vi "AfterZeroSpreadColor-V2.2.vi"(4 "BackMap":i32[][](array[numeric]), 5 "WhichPlayer":i32, 6 "Position":i32[][](array[numeric])=[[0, 1], [1, 0]]) -> (0 "col":i32, 1 "row":i32, 2 "Numeric":dbl)   [LabVIEW 2014]
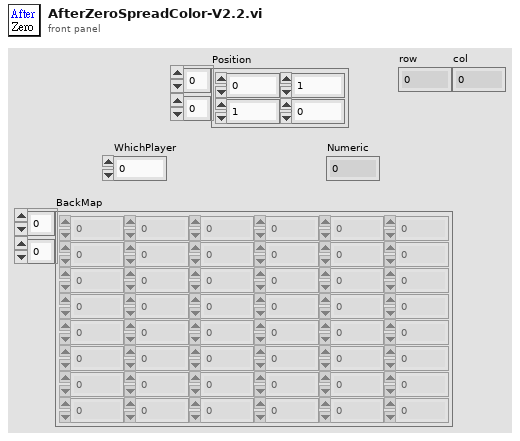
[diagram p1: front panel]
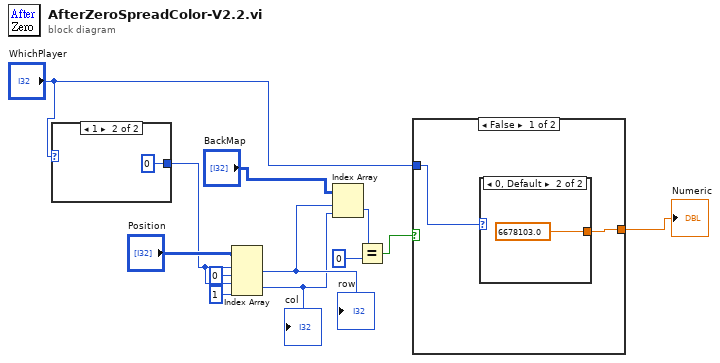
[diagram p0: block diagram]
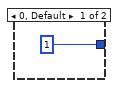
[diagram p2: hidden frame]
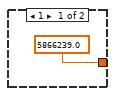
[diagram p3: hidden frame]
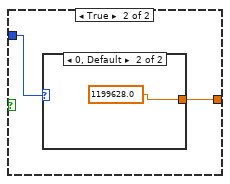
[diagram p4: hidden frame]
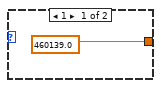
[diagram p5: hidden frame]
diagram:
  n1 = case shown="1" "WhichPlayer" {
    tunnel: [1 0] -> w5
    frame 0, Default {
    }
    frame 1 {
    }
  }
  n2 = Index Array(array="Position", index (row) #1=w5, index (col) #1=0 ("disabled index (col)"), index (row) #2=w5, index (col) #2=1 ("disabled index (col)")) -> (element #1=w2:i32, element #2=w1:i32)
  "row" <- w2
  "col" <- w1
  n3 = Index Array(array="BackMap", index (row)=w2, index (col)=w1) -> (element=w12:i32)
  n4 = Equal?(x=w12, y=0) -> (x = y?=w10:bool)
  n5 = case shown="False" w10 {
    tunnel: [w16 w20] -> w8
    tunnel: "WhichPlayer" -> [w15 w19]
    frame False {
      n6 = case shown="0, Default" w15 {
        tunnel: [5866239.0 6678103.0] -> w16
        frame 1 {
        }
        frame 0, Default {
        }
      }
    }
    frame True {
      n7 = case shown="0, Default" w19 {
        tunnel: [460139.0 1199628.0] -> w20
        frame 1 {
        }
        frame 0, Default {
        }
      }
    }
  }
  "Numeric" <- w8
